vi "scan harm.vi"() -> ()   [LabVIEW 2019]
uses:
  SubVI/ctl/config.ctl
  <vilib>/NI/Modbus Library/API/Master/Modbus Master.lvclass
  SubVI/ctl/initialize.ctl
  SubVI/ctl/Instrument.ctl
  SubVI/ctl/limit.ctl
  SubVI/ctl/warning.ctl
  SubVI/ctl/Instrument Type.ctl
  SubVI/ctl/335 state.ctl
  SubVI/ctl/9T mag field stauts.ctl
  C:/Users/fuyang/Desktop/postdoctor/labview/labview-measure/lib/QDInstrument.dll
  lib/QDInstrument.dll
  SubVI/ctl/Gating type.ctl
  SubVI/SubVI.lvlib
  <vilib>/measure/NI_MABase.lvlib
  SubVI/nematic/Copy of StrainCell.lvlib
panel:
  out "Waveform Graph 2":waveform(dbl)(graph)
  out "Waveform Graph":waveform(dbl)(graph)
  out "R 2":cluster{i32[], dbl[]}(graph) caption="R"
  out "θ 2":cluster{i32[], dbl[]}(graph) caption="θ"
  out "freq 2":cluster{i32[], dbl[]}(graph) caption="FREQ"
  out "freq":cluster{i32[], dbl[]}(graph) caption="FREQ"
  out "θ":cluster{i32[], dbl[]}(graph)
  out "R":cluster{i32[], dbl[]}(graph)
  in  "簇":T1={"initialize"=enum."SR830", "6221"={"6221 Resource"="GPIB1::10::INSTR", "Delta status"=FALSE, "电流|RMS(A)"=0.0}, "SR830+6221"={"source"=4, "Current(A)"=0.0, "阻抗(Ohm)"=0.0001, "SR830 1"=TRUE, "SR830 2"=TRUE, "SR830 3"=FALSE, "SR830 4"=FALSE, "VISA 1"="GPIB0::4::INSTR", "VISA 2"="GPIB0::3::INSTR", "VISA 3"="", "VISA 4"="", "Reserve 1"=0, "Reserve 2"=-1, "Reserve 3"=-1, "Reserve 4"=-1, "Sensitivity 1"=-1, "Sensitivity 2"=-1, "Sensitivity 3"=-1, "Sensitivity 4"=-1, "量程入 1"=0, "量程入 2"=0, "量程入 3"=0, "量程入 4"=0}, "2400"={"2400"=FALSE, "VISA"="", "Output Level (0)"=1e-05, "Compliance  Level (0.1)"=10.0, "ch"=[]}, "ch"={"ch"=[], "current"=[], "change?"=[], "holding current\nwhen change ch?"=FALSE, "current offset"=[]}, "Instrument"={"limit"={"Field limit"=0.0, "Field rate limit"=3.0, "Temp limit"=1.0, "Temp low limit"=0.0, "Temp rate limit "=0.0}, "genarl"={"行数"=refnum, "编辑列表框？"=refnum, "列表框"=refnum, "camg 振荡状态"=refnum, "Aborting"=refnum, "数据文件"=refnum, "warning"=refnum, "vi路径"="GPIB0::24::INSTR", "Instrument Type"=enum."PPMS-Rotate"}, "cmag"={"TM620"="GPIB0::24::INSTR", "M24C Resource"="GPIB0::24::INSTR", "4G supply"="GPIB0::24::INSTR", "Temp Status 24C"=refnum, "Temp"=refnum, "9T信号"=refnum, "4g supply status"=refnum, "in-plane"="", "out-plane"="", "in-plane signal"=FALSE, "out-plane signal"=FALSE, "in plane 信号"=refnum, "pzt volt"=refnum, "camg Rate"=refnum}, "lengtou2"={"750 visa"="", "750 rotate"="", "semaphore 340"=refnum, "semaphore 750"=refnum, "750 field status"=refnum, "Input (0:A) 340"=0, "340 Resource"="GPIB0::14::INSTR", "340 Status"=refnum, "Input (0:B) 340"=1, "Loop (0: 1)"=0, "Loop (1: 1)"=0, "TCP master instance"=refnum}, "lengtou"={"TCP master instance"=refnum, "335 Status"=refnum, "335 Resource "="GPIB0::24::INSTR", "Input (0:A) 335"=0, "Input (0:B) 335"=1, "Heater Output (1:1) 335"=1, "semaphore 335"=refnum}, "325 for test"={"quantum design"=refnum, "semaphore 325"=refnum, "325 Resource "="GPIB0::13::INSTR", "Input (0:A) 325"=0, "Heater Output (1:1) 325"=1, "325 Status"=refnum}}, "2614B"={"2614B chA"=FALSE, "2614B chB"=FALSE, "VISA"=""}, "33522b"={"33522b resource name"="", "零电压"=0.0, "最大电压"=148.0, "间隔"=4.0, "最小电压"=-48.0, "loop"=0.0, "压电陶瓷电压(Vpp)"=0.0}, "gating type"=enum."2614(daul)", "层数"=0, "行数"=0, "是否处理"=[], "current 2"=[], "StrainCell"={"RP100 resource name"="COM8", "E4980 resource name"="GPIB0::10::INSTR", "RP100 Reset ?(True)"=FALSE, "Voltage1(V)"=0.0, "Voltage2(V)"=0.0, "interval"=4.0, "slew(V/s)"=1.0}} {"Instrument"."325 for test"."Heater Output (1:1) 325" items=["1"=1, "2"=2]; "Instrument"."325 for test"."Input (0:A) 325" items=["A", "B"]; "Instrument"."lengtou"."Heater Output (1:1) 335" items=["1"=1, "2"=2]; "Instrument"."lengtou"."Input (0:B) 335" items=["A", "B"]; "Instrument"."lengtou"."Input (0:A) 335" items=["A", "B"]; "Instrument"."lengtou2"."Loop (1: 1)" items=["1", "2"]; "Instrument"."lengtou2"."Loop (0: 1)" items=["1", "2"]; "Instrument"."lengtou2"."Input (0:B) 340" items=["A", "B", "C", "D"]; "Instrument"."lengtou2"."Input (0:A) 340" items=["A", "B", "C", "D"]; "SR830+6221"."Sensitivity 4" items=["Auto Gain"=-1, "2 nV/fA"=0, "5 nV/fA"=1, "10 nV/fA"=2, "20 nV/fA"=3, "50 nV/fA"=4, "100 nV/fA"=5, "200 nV/fA"=6, "500 nV/fA"=7, "1 uV/pA"=8, "2 uV/pA"=9, "5 uV/pA"=10, "10 uV/pA"=11, "20 uV/pA"=12, "50 uV/pA"=13, "100 uV/pA"=14, "200 uV/pA"=15, "500 uV/pA"=16, "1 mV/nA"=17, "2 mV/nA"=18, "5 mV/nA"=19, "10 mV/nA"=20, "20 mV/nA"=21, "50 mV/nA"=22, "100 mV/nA"=23, "200 mV/nA"=24, "500 mV/mA"=25, "1 V/uA"=26]; "SR830+6221"."Sensitivity 3" items=["Auto Gain"=-1, "2 nV/fA"=0, "5 nV/fA"=1, "10 nV/fA"=2, "20 nV/fA"=3, "50 nV/fA"=4, "100 nV/fA"=5, "200 nV/fA"=6, "500 nV/fA"=7, "1 uV/pA"=8, "2 uV/pA"=9, "5 uV/pA"=10, "10 uV/pA"=11, "20 uV/pA"=12, "50 uV/pA"=13, "100 uV/pA"=14, "200 uV/pA"=15, "500 uV/pA"=16, "1 mV/nA"=17, "2 mV/nA"=18, "5 mV/nA"=19, "10 mV/nA"=20, "20 mV/nA"=21, "50 mV/nA"=22, "100 mV/nA"=23, "200 mV/nA"=24, "500 mV/mA"=25, "1 V/uA"=26]; "SR830+6221"."Sensitivity 1" items=["Auto Gain"=-1, "2 nV/fA"=0, "5 nV/fA"=1, "10 nV/fA"=2, "20 nV/fA"=3, "50 nV/fA"=4, "100 nV/fA"=5, "200 nV/fA"=6, "500 nV/fA"=7, "1 uV/pA"=8, "2 uV/pA"=9, "5 uV/pA"=10, "10 uV/pA"=11, "20 uV/pA"=12, "50 uV/pA"=13, "100 uV/pA"=14, "200 uV/pA"=15, "500 uV/pA"=16, "1 mV/nA"=17, "2 mV/nA"=18, "5 mV/nA"=19, "10 mV/nA"=20, "20 mV/nA"=21, "50 mV/nA"=22, "100 mV/nA"=23, "200 mV/nA"=24, "500 mV/mA"=25, "1 V/uA"=26]; "SR830+6221"."Sensitivity 2" items=["Auto Gain"=-1, "2 nV/fA"=0, "5 nV/fA"=1, "10 nV/fA"=2, "20 nV/fA"=3, "50 nV/fA"=4, "100 nV/fA"=5, "200 nV/fA"=6, "500 nV/fA"=7, "1 uV/pA"=8, "2 uV/pA"=9, "5 uV/pA"=10, "10 uV/pA"=11, "20 uV/pA"=12, "50 uV/pA"=13, "100 uV/pA"=14, "200 uV/pA"=15, "500 uV/pA"=16, "1 mV/nA"=17, "2 mV/nA"=18, "5 mV/nA"=19, "10 mV/nA"=20, "20 mV/nA"=21, "50 mV/nA"=22, "100 mV/nA"=23, "200 mV/nA"=24, "500 mV/mA"=25, "1 V/uA"=26]; "SR830+6221"."Reserve 4" items=["Auto Reserve"=-1, "High Reserve"=0, "Normal"=1, "Low Noise"=2]; "SR830+6221"."Reserve 3" items=["Auto Reserve"=-1, "High Reserve"=0, "Normal"=1, "Low Noise"=2]; "SR830+6221"."Reserve 2" items=["Auto Reserve"=-1, "High Reserve"=0, "Normal"=1, "Low Noise"=2]; "SR830+6221"."Reserve 1" items=["Auto Reserve"=-1, "High Reserve"=0, "Normal"=1, "Low Noise"=2]; "SR830+6221"."source" items=["SR830 1", "SR830 2", "SR830 3", "SR830 4"]}
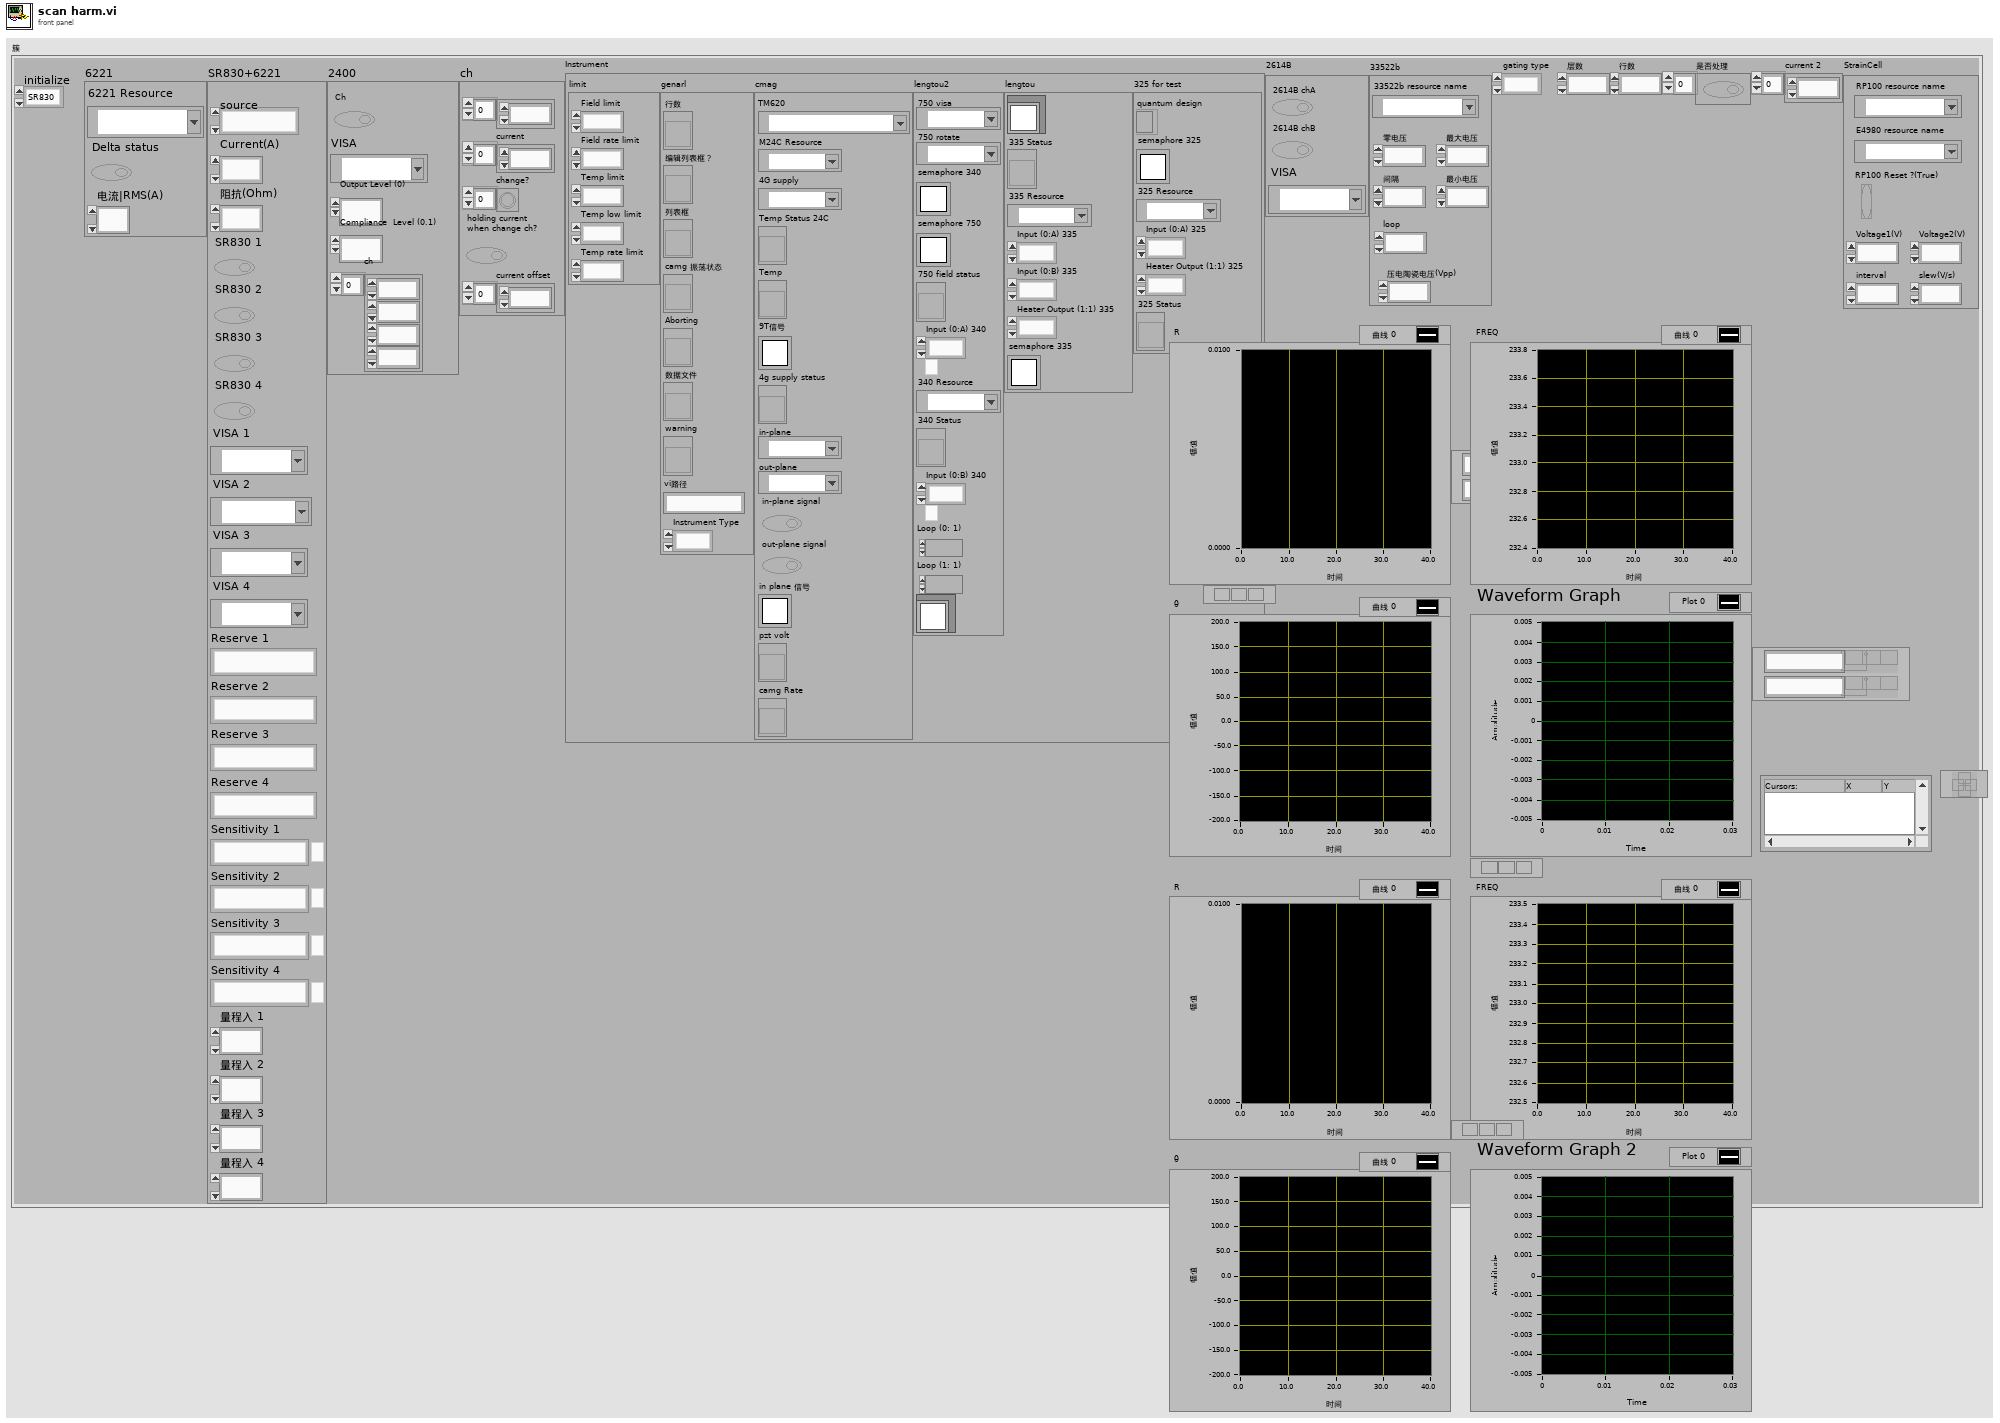
[diagram p1: front panel]
types:
  T1 = typedef "config.ctl" = cluster{"initialize":T2, "6221":cluster{"6221 Resource":refnum<visa-resource-name>, "Delta status":bool, "电流|RMS(A)":dbl}, "SR830+6221":cluster{"source":u16, "Current(A)":dbl, "阻抗(Ohm)":dbl, "SR830 1":bool, "SR830 2":bool, "SR830 3":bool, "SR830 4":bool, "VISA 1":refnum<visa-resource-name>, "VISA 2":refnum<visa-resource-name>, "VISA 3":refnum<visa-resource-name>, "VISA 4":refnum<visa-resource-name>, "Reserve 1":i16, "Reserve 2":i16, "Reserve 3":i16, "Reserve 4":i16, "Sensitivity 1":i16, "Sensitivity 2":i16, "Sensitivity 3":i16, "Sensitivity 4":i16, "量程入 1":i32, "量程入 2":i32, "量程入 3":i32, "量程入 4":i32}, "2400":cluster{"2400":bool, "VISA":refnum<visa-resource-name>, "Output Level (0)":dbl, "Compliance  Level (0.1)":dbl, "ch":i32[]}, "ch":cluster{"ch":i32[], "current":dbl[], "change?":bool[], "holding current\nwhen change ch?":bool, "current offset":dbl[]}, "Instrument":T3, "2614B":cluster{"2614B chA":bool, "2614B chB":bool, "VISA":refnum<visa-resource-name>}, "33522b":cluster{"33522b resource name":refnum<visa-resource-name>, "零电压":dbl, "最大电压":dbl, "间隔":dbl, "最小电压":dbl, "loop":dbl, "压电陶瓷电压(Vpp)":dbl}, "gating type":T7, "层数":i32, "行数":i32, "是否处理":bool[], "current 2":dbl[], "StrainCell":cluster{"RP100 resource name":refnum<visa-resource-name>, "E4980 resource name":refnum<visa-resource-name>, "RP100 Reset ?(True)":bool, "Voltage1(V)":dbl, "Voltage2(V)":dbl, "interval":dbl, "slew(V/s)":dbl}}
  T2 = typedef "initialize.ctl" = enum16{"SR830", "keithley6221-SR830", "Delta", "Delta-tunnelling", "keithley6221-2182-DC", "PZT", "StrainCell", "4200"}
  T3 = typedef "Instrument.ctl" = cluster{"limit":T4, "genarl":cluster{"行数":refnum<vi>, "编辑列表框？":refnum<vi>, "列表框":refnum<vi>, "camg 振荡状态":refnum<vi>, "Aborting":refnum<vi>, "数据文件":refnum<vi>, "warning":refnum<vi>, "vi路径":string, "Instrument Type":T5}, "cmag":cluster{"TM620":refnum<visa-resource-name>, "M24C Resource":refnum<visa-resource-name>, "4G supply":refnum<visa-resource-name>, "Temp Status 24C":refnum<vi>, "Temp":refnum<vi>, "9T信号":T6, "4g supply status":refnum<vi>, "in-plane":refnum<visa-resource-name>, "out-plane":refnum<visa-resource-name>, "in-plane signal":bool, "out-plane signal":bool, "in plane 信号":T6, "pzt volt":refnum<vi>, "camg Rate":refnum<vi>}, "lengtou2":cluster{"750 visa":refnum<visa-resource-name>, "750 rotate":refnum<visa-resource-name>, "semaphore 340":T6, "semaphore 750":T6, "750 field status":refnum<vi>, "Input (0:A) 340":u16, "340 Resource":refnum<visa-resource-name>, "340 Status":refnum<vi>, "Input (0:B) 340":u16, "Loop (0: 1)":u16, "Loop (1: 1)":u16, "TCP master instance":refnum<class "Modbus Master.lvclass">}, "lengtou":cluster{"TCP master instance":refnum<class "Modbus Master.lvclass">, "335 Status":refnum<vi>, "335 Resource ":refnum<visa-resource-name>, "Input (0:A) 335":u16, "Input (0:B) 335":u16, "Heater Output (1:1) 335":u16, "semaphore 335":T6}, "325 for test":cluster{"quantum design":refnum<k24>, "semaphore 325":T6, "325 Resource ":refnum<visa-resource-name>, "Input (0:A) 325":u16, "Heater Output (1:1) 325":u16, "325 Status":refnum<vi>}}
  T4 = typedef "limit.ctl" = cluster{"Field limit":dbl, "Field rate limit":dbl, "Temp limit":dbl, "Temp low limit":dbl, "Temp rate limit ":dbl}
  T5 = typedef "Instrument Type.ctl" = enum16{"PPMS", "VersaLab", "DynaCool", "SVSM", "PPMS-Rotate", "Lakeshore335", "2T cmag", "9T mag old", "9T cmag", "9T cmag DAC", "9T cmag rotate", "test"}
  T6 = typedef "Semaphore RefNum" = refnum<k1>
  T7 = typedef "Gating type.ctl" = enum32{"null", "2614(daul)", "2400", "6517B"}
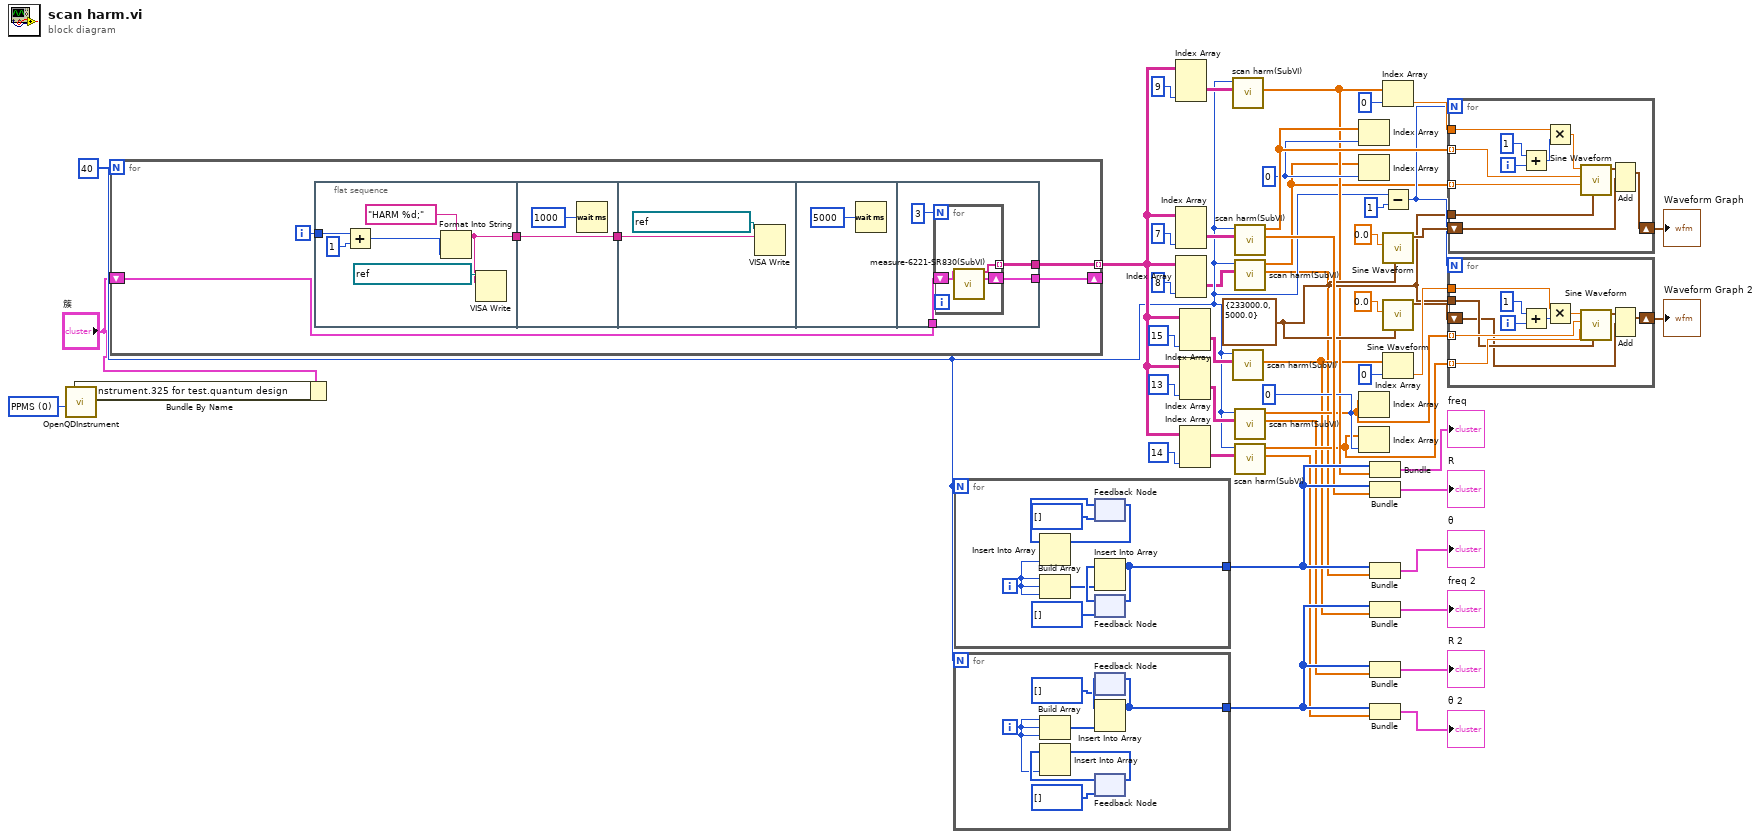
[diagram p0: block diagram]
diagram:
  w19 = cluster{"Fs":dbl, "#s":dbl} {"Fs"=233000.0, "#s"=5000.0} ("sampling info")
  w23 = 0 ("index")
  w27 = 0 ("index")
  w31 = 0 items=["PPMS", "VersaLab", "DynaCool", "SVSM"] ("Instrument Type")
  w8 = 40
  n1 = call "OpenQDInstrument.vi"("Instrument Type"=w31) -> ("Instrument Ref"=w1:refnum<k24>)  [unwired: 7 in, 1 out]
  n2 = Bundle By Name(cluster="簇", "Instrument.325 for test.quantum design"=w1) -> ()  [unwired: 1 out]
  n3 = for {
    N: w8 -> [_]
    tunnel: [w55] -> w32 mode=indexing
    shift-right: [w51] -> _
    shift-left: "簇" -> [w52]
    i -> [w56]
    n4 = flat-sequence {
      tunnel: w56 -> [w60]
      tunnel: [w57] -> w54
      tunnel: w54 -> [w64]
      tunnel: [w64] -> w53
      tunnel: w53 -> [w66]
      tunnel: [w70] -> w55
      tunnel: w52 -> [w69]
      tunnel: [w68] -> w51
      frame #0 {
        n5 = Add(x=w60, y=1) -> (x+y=w58:i32)
        n6 = Format Into String(format string="HARM %d;", w58) -> (resulting string=w57:string)  [unwired: 2 in, 1 out]
        n7 = VISA Write(VISA resource name=refnum<visa-resource-name> "GPIB0::3::INSTR", write buffer=w57) -> ()  [unwired: 1 in, 3 out]
      }
      frame #1 {
        n8 = Wait (ms)(milliseconds to wait=u32 1000) -> ()  [unwired: 1 out]
      }
      frame #2 {
        n9 = VISA Write(VISA resource name=refnum<visa-resource-name> "GPIB0::4::INSTR", write buffer=w66) -> ()  [unwired: 1 in, 3 out]
      }
      frame #3 {
        n10 = Wait (ms)(milliseconds to wait=u32 5000) -> ()  [unwired: 1 out]
      }
      frame #4 {
        n11 = for {
          N: 3 -> [_]
          tunnel: [w74] -> w70 mode=indexing
          shift-right: [w73] -> w68
          shift-left: w69 -> [w72]
          n12 = call "measure-6221-SR830(SubVI).vi"("输入簇"=w72) -> ("输出数组"=w74:string[], "输出簇"=w73:T1)  [unwired: 12 in, 1 out]
        }
      }
    }
  }
  n13 = for {
    N: w8 -> [_]
    tunnel: [w80] -> w45
    i -> [w75]
    n14 = Build Array(w75, w75, w75) -> (w79:i32[])
    n15 = feedback #1(i32[] []) -> (w76:i32[])
    n16 = Insert Into Array(array=w76, new element=w75) -> (w78:i32[])  [unwired: 1 in]
    n17 = feedback-in #1(w78) -> ()
    n18 = feedback #2(i32[] []) -> (w82:i32[])
    n19 = Insert Into Array(array=w82, new element=w79) -> (w80:i32[])  [unwired: 1 in]
    n20 = feedback-in #2(w80) -> ()
  }
  n21 = for {
    N: w8 -> [_]
    tunnel: [w88] -> w37
    i -> [w83]
    n22 = Build Array(w83, w83, w83) -> (w87:i32[])
    n23 = feedback #3(i32[] []) -> (w90:i32[])
    n24 = Insert Into Array(array=w90, new element=w87) -> (w88:i32[])  [unwired: 1 in]
    n25 = feedback-in #3(w88) -> ()
    n26 = feedback #4(i32[] []) -> (w84:i32[])
    n27 = Insert Into Array(array=w84, new element=w83) -> (w86:i32[])  [unwired: 1 in]
    n28 = feedback-in #4(w86) -> ()
  }
  n29 = Index Array(array=w32, index (dim 2)=9 ("索引 (列)")) -> (element=w18:string[][])  [unwired: 2 in]
  n30 = Index Array(array=w32, index (dim 2)=7 ("索引 (列)")) -> (element=w47:string[][])  [unwired: 2 in]
  n31 = Index Array(array=w32, index (dim 2)=8 ("禁用的索引 (列)")) -> (element=w7:string[][])  [unwired: 2 in]
  n32 = Index Array(array=w32, index (dim 2)=15 ("索引 (列)")) -> (element=w10:string[][])  [unwired: 2 in]
  n33 = Index Array(array=w32, index (dim 2)=13 ("索引 (列)")) -> (element=w13:string[][])  [unwired: 2 in]
  n34 = Index Array(array=w32, index (dim 2)=14 ("禁用的索引 (列)")) -> (element=w16:string[][])  [unwired: 2 in]
  n35 = call "scan harm(SubVI).vi"("输出数组"=w18, "Numeric"=w8) -> ("Array 2"=w17:dbl[])  [unwired: 8 in, 1 out]
  n36 = call "scan harm(SubVI).vi"("输出数组"=w10, "Numeric"=w8) -> ("Array 2"=w9:dbl[])  [unwired: 8 in, 1 out]
  n37 = call "scan harm(SubVI).vi"("输出数组"=w47, "Numeric"=w8) -> ("Array 2"=w42:dbl[], "Array"=w29:dbl[])  [unwired: 8 in]
  n38 = call "scan harm(SubVI).vi"("输出数组"=w7, "Numeric"=w8) -> ("Array 2"=w5:dbl[], "Array"=w6:dbl[])  [unwired: 8 in]
  n39 = call "scan harm(SubVI).vi"("输出数组"=w13, "Numeric"=w8) -> ("Array 2"=w11:dbl[], "Array"=w12:dbl[])  [unwired: 8 in]
  n40 = call "scan harm(SubVI).vi"("输出数组"=w16, "Numeric"=w8) -> ("Array 2"=w14:dbl[], "Array"=w15:dbl[])  [unwired: 8 in]
  n41 = Index Array(array=w29, index=w27) -> ()  [unwired: 1 out]
  n42 = Index Array(array=w6, index=w27) -> ()  [unwired: 1 out]
  n43 = Index Array(array=w12, index=w23) -> ()  [unwired: 1 out]
  n44 = Index Array(array=w15, index=w23) -> ()  [unwired: 1 out]
  n45 = Bundle(w45, "Array 2"=w17) -> (→"freq":cluster{i32[], "Array 2":dbl[]})  [unwired: 1 in]
  n46 = Bundle(w45, "Array 2"=w42) -> (→"R":cluster{i32[], "Array 2":dbl[]})  [unwired: 1 in]
  n47 = Bundle(w45, "Array 2"=w5) -> (→"θ":cluster{i32[], "Array 2":dbl[]})  [unwired: 1 in]
  n48 = Bundle(w37, "Array 2"=w9) -> (→"freq 2":cluster{i32[], "Array 2":dbl[]})  [unwired: 1 in]
  n49 = Bundle(w37, "Array 2"=w11) -> (→"R 2":cluster{i32[], "Array 2":dbl[]})  [unwired: 1 in]
  n50 = Bundle(w37, "Array 2"=w14) -> (→"θ 2":cluster{i32[], "Array 2":dbl[]})  [unwired: 1 in]
  n51 = Index Array(array=w17, index=0 ("索引")) -> (element=w28:dbl)
  n52 = Subtract(x=w8, y=1) -> (x-y=w21:i32)
  n53 = call <vilib>:"Sine Waveform.vi"("sampling info"=w19, "amplitude"=0.0) -> ("signal out"=w26:waveform(dbl))  [unwired: 8 in, 1 out]
  n54 = call <vilib>:"Sine Waveform.vi"("sampling info"=w19, "amplitude"=0.0) -> ("signal out"=w20:waveform(dbl))  [unwired: 8 in, 1 out]
  n55 = Index Array(array=w9, index=0 ("索引")) -> (element=w22:dbl)
  n56 = for {
    N: w21 -> [_]
    tunnel: w29 -> [w101] mode=indexing
    tunnel: w6 -> [w100] mode=indexing
    tunnel: w28 -> [w99]
    tunnel: w19 -> [w93]
    shift-right: [w92] -> w25
    shift-left: w26 -> [w91]
    i -> [w98]
    n57 = Add(x=1, y=w98) -> (x+y=w96:i32)
    n58 = Multiply(x=w99, y=w96) -> (x*y=w95:dbl)
    n59 = call <vilib>:"Sine Waveform.vi"("sampling info"=w93, "phase"=w100, "amplitude"=w101, "frequency"=w95) -> ("signal out"=w94:waveform(dbl))  [unwired: 6 in, 1 out]
    n60 = Add(1:w91, 2:w94) -> (0:w92:waveform(dbl))  [unwired: 1 in, 1 out]
  }
  "Waveform Graph" <- w25
  n61 = for {
    N: w21 -> [_]
    tunnel: w12 -> [w112] mode=indexing
    tunnel: w15 -> [w111] mode=indexing
    tunnel: w22 -> [w110]
    tunnel: w19 -> [w104]
    shift-right: [w102] -> w24
    shift-left: w20 -> [w103]
    i -> [w109]
    n62 = Add(x=1, y=w109) -> (x+y=w107:i32)
    n63 = Multiply(x=w110, y=w107) -> (x*y=w106:dbl)
    n64 = call <vilib>:"Sine Waveform.vi"("sampling info"=w104, "phase"=w111, "amplitude"=w112, "frequency"=w106) -> ("signal out"=w105:waveform(dbl))  [unwired: 6 in, 1 out]
    n65 = Add(1:w103, 2:w105) -> (0:w102:waveform(dbl))  [unwired: 1 in, 1 out]
  }
  "Waveform Graph 2" <- w24
